vi "Write Qsh.vi"(8 "error in (no error)":errorcluster, 10 "Qsh":dbl, 11 "DMA in":refnum<class "DMA.lvclass">) -> (0 "error out":errorcluster, 3 "DMA out":refnum<class "DMA.lvclass">)   [LabVIEW 2015, in "DMA.lvclass"]
doc: "Assume that the input is in lpm. We will convert this to m3/s and store this value."
uses:
  DMA.lvclass
  DMA.lvclass/DMA.ctl
  Conversion Constants.vi
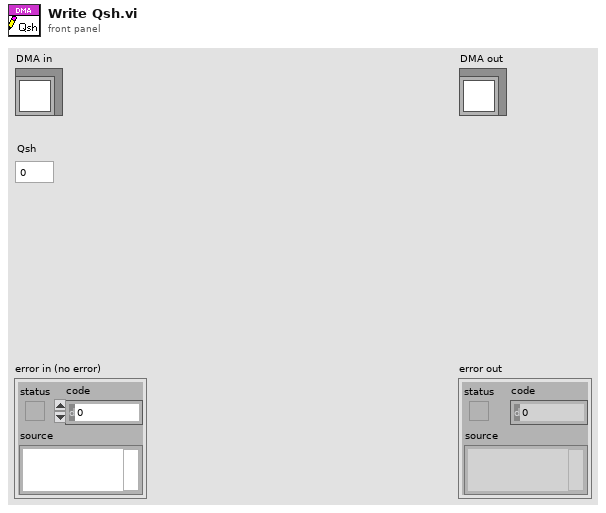
[diagram p1: front panel]
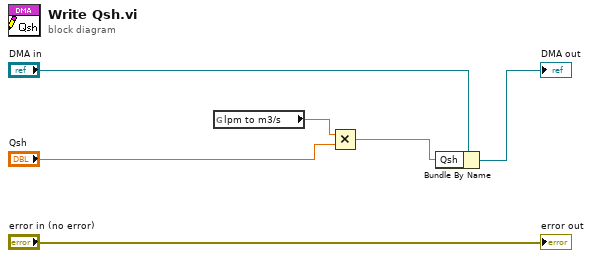
[diagram p0: block diagram]
diagram:
  n1 = global read "Conversion Constants.vi" "lpm to m3/s"() -> (w2:dbl)
  n2 = Multiply(x=w2, y="Qsh") -> (x*y=w1:dbl)
  n3 = Bundle By Name(cluster="DMA in", "Qsh"=w1) -> (→"DMA out":refnum<class "DMA.lvclass">)
  "error out" <- "error in (no error)"
